vi "APS get sscnet servo param.vi"(6 "Para_Dat2":i32, 7 "Para_No2":i32, 8 "error in (no error)":errorcluster caption="错误输入（无错误）", 9 "Para_Dat1":i32, 10 "Para_No1":i32, 11 "Axis_ID":i32) -> (0 "error out":errorcluster caption="错误输出", 1 "Para_Dat1 out":i32, 3 "function return":i32, 4 "Para_Dat2 out":i32)   [LabVIEW 2011, in "APS168.lvlib"]
doc: "I32 FNTYPE APS_get_sscnet_servo_param( I32 Axis_ID, I32 Para_No1, I32 *Para_Dat1, I32 Para_No2, I32 *Para_Dat2 );"
uses:
  APS168.lvlib
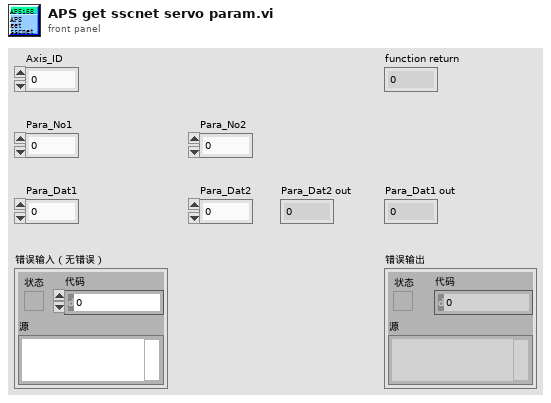
[diagram p1: front panel]
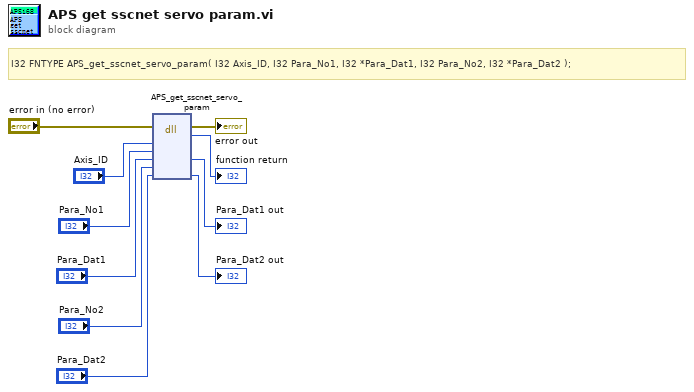
[diagram p0: block diagram]
diagram:
  # "I32 FNTYPE APS_get_sscnet_servo_param( I32 Axis_ID, I32 Para_No1, I32 *Para_Dat1, I32 Para_No2, I32 *Para_Dat2 );"
  n1 = dll-call lib="PTH1Labs E软件ADLINK 204CAPS_1_7_1_LIB line 连续运动204APS168.*" fn="APS_get_sscnet_servo_param"(error in="error in (no error)", "Axis_ID"="Axis_ID", "Para_No1"="Para_No1", "Para_Dat1"="Para_Dat1", "Para_No2"="Para_No2", "Para_Dat2"="Para_Dat2") -> (error out=→"error out":errorcluster, →"function return":i32, "Para_Dat1"=→"Para_Dat1 out":i32, "Para_Dat2"=→"Para_Dat2 out":i32)  [unwired: 5 in, 1 out]
